vi "Run.vi"(8 "error in (no error)":errorcluster, 9 "s on last turn":dbl, 10 "Maze (0: Empty, -1: Enemy. >0: Teammate":i32[][](array[numeric]), 11 "Attack in":refnum<class "Net Attack.lvclass">) -> (0 "error out":errorcluster, 1 "Direction":T1, 2 "Action":T2, 3 "Attack out":refnum<class "Net Attack.lvclass">, 4 "Replicated":refnum<class "Square.lvclass">)   [LabVIEW 2014, in "Net Attack.lvclass"]
uses:
  Net Attack.lvclass
  SquareBattle Arena/Action Enum.ctl
  SquareBattle Arena/Direction Enum.ctl
  Square.lvclass
  Net Attack.lvclass/Net Attack.ctl
  SquareBattle Arena/SquareBattle Arena.lvclass
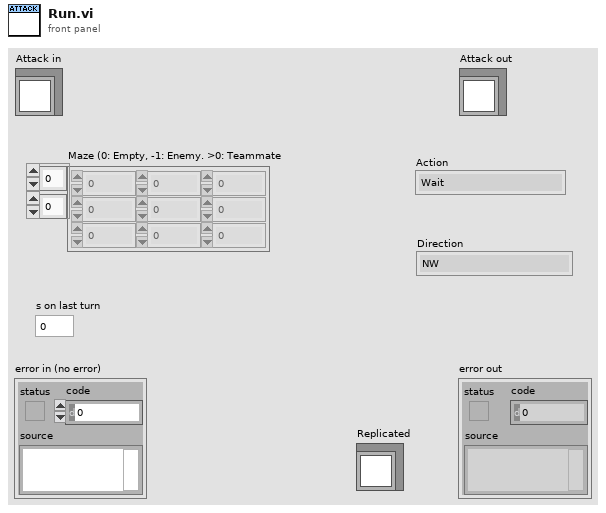
[diagram p1: front panel]
types:
  T1 = typedef "SquareBattle Arena.lvlib/SquareBattle Arena.lvclass/Direction Enum.ctl" = enum16{"NW", "N", "NE", "E", "SE", "S", "SW", "W"}
  T2 = typedef "SquareBattle Arena.lvlib/SquareBattle Arena.lvclass/Action Enum.ctl" = enum16{"Wait", "Move", "Attack", "Replicate"}
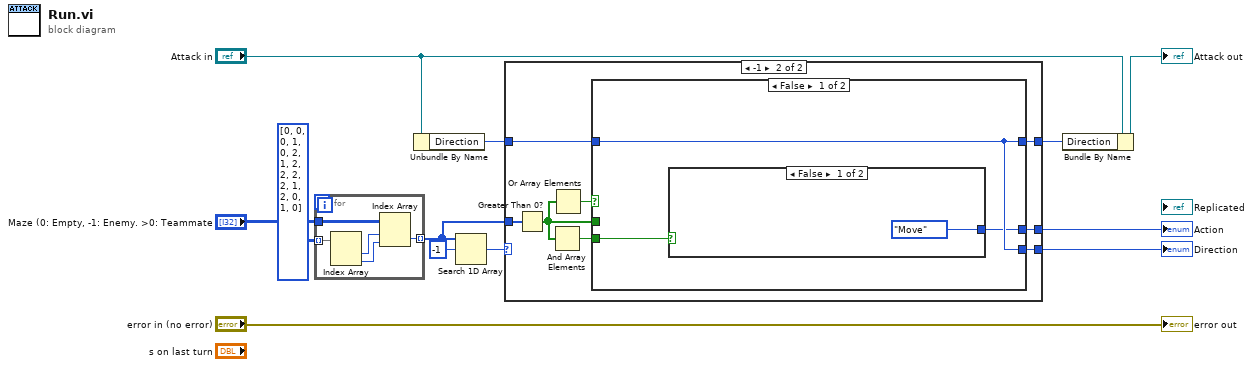
[diagram p0: block diagram]
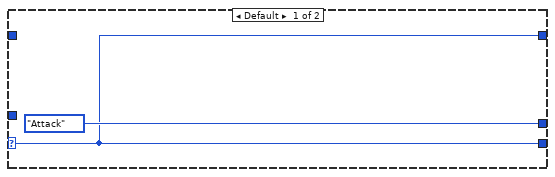
[diagram p2: hidden frame]
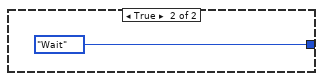
[diagram p3: hidden frame]
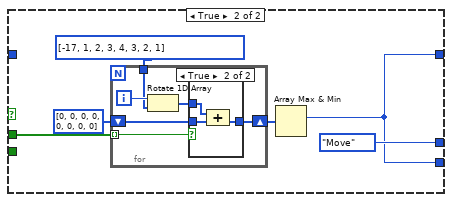
[diagram p4: hidden frame]
diagram:
  n1 = for {
    tunnel: "Maze (0: Empty, -1: Enemy. >0: Teammate" -> [w17]
    tunnel: i32[][] [[0, 0], [0, 1], [0, 2], [1, 2], [2, 2], [2, 1], [2, 0], [1, 0]] -> [w16] mode=indexing
    tunnel: [w13] -> w5 mode=indexing
    n2 = Index Array(array=w16) -> (element #1=w15:i32, element #2=w14:i32)  [unwired: 2 in]
    n3 = Index Array(array=w17, index (row)=w15, index (col)=w14) -> (element=w13:i32)
  }
  n4 = Unbundle By Name("Attack in") -> ("Direction"=w4:T1)
  n5 = Search 1D Array(1D array=w5, element=-1) -> (index of element=w6:i32)  [unwired: 1 in]
  n6 = case shown="-1" w6 {
    selector: w6 -> [w18 _]
    tunnel: [w18 w24] -> w2
    tunnel: [Action_Enum."Attack" ("Action") w23] -> w3
    tunnel: w4 -> [_ w26]
    tunnel: w5 -> [_ w27]
    tunnel: [w18 w25] -> w1
    frame Default {
    }
    frame -1 {
      n7 = Greater Than 0?(x=w27) -> (x > 0?=w22:bool[])
      n8 = And Array Elements(Boolean array=w22) -> (logical AND=w21:bool)
      n9 = Or Array Elements(Boolean array=w22) -> (logical OR=w20:bool)
      n10 = case shown="False" w20 {
        tunnel: w26 -> [w30 _]
        tunnel: [w30 w33] -> w25
        tunnel: [w30 w33] -> w24
        tunnel: [w28 Action_Enum."Move" ("Action")] -> w23
        tunnel: w22 -> [_ w37]
        tunnel: w21 -> [w29 _]
        frame False {
          n11 = case shown="False" w29 {
            tunnel: [Action_Enum."Move" ("t") Action_Enum."Wait" ("t")] -> w28
            frame False {
            }
            frame True {
            }
          }
        }
        frame True {
          n12 = for {
            tunnel: w37 -> [w42] mode=indexing
            tunnel: i32[] [-17, 1, 2, 3, 4, 3, 2, 1] -> [w43]
            shift-right: [w40] -> w34
            shift-left: i32[] [0, 0, 0, 0, 0, 0, 0, 0] -> [w39]
            i -> [w44]
            n13 = Rotate 1D Array(1:w43, 2:w44) -> (0:w41:i32[])
            n14 = case shown="True" w42 {
              tunnel: w41 -> [_ w48]
              tunnel: [w45 w47] -> w40
              tunnel: w39 -> [w45 w46]
              frame False {
              }
              frame True {
                n15 = Compound Arithmetic op=ADD(w48, w46) -> (w47:i32[])
              }
            }
          }
          n16 = Array Max & Min(array=w34) -> (max index (indices)=w33:i32)  [unwired: 3 out]
        }
      }
    }
  }
  "Action" <- w3
  "Direction" <- w2
  n17 = Bundle By Name(cluster="Attack in", "Direction"=w1) -> (→"Attack out":refnum<class "Net Attack.lvclass">)
  "error out" <- "error in (no error)"
